vi "createTempControllerFrontEndEvents.vi"(8 "error in (no error)":errorcluster, 11 "CameraEventsManger.lvclass in":refnum<class "CameraEventsManger.lvclass">) -> (0 "error out":errorcluster, 2 "tempControllerFrontEndEvents":T1, 3 "CameraEventsManger.lvclass out":refnum<class "CameraEventsManger.lvclass">)   [LabVIEW 2011, in "Tools.lvlib" / "Settings.lvlib" / "CameraEventsManger.lvclass"]
uses:
  CameraEventsManger.lvclass
  CameraEventsManger.lvclass/CameraEventsManger.ctl
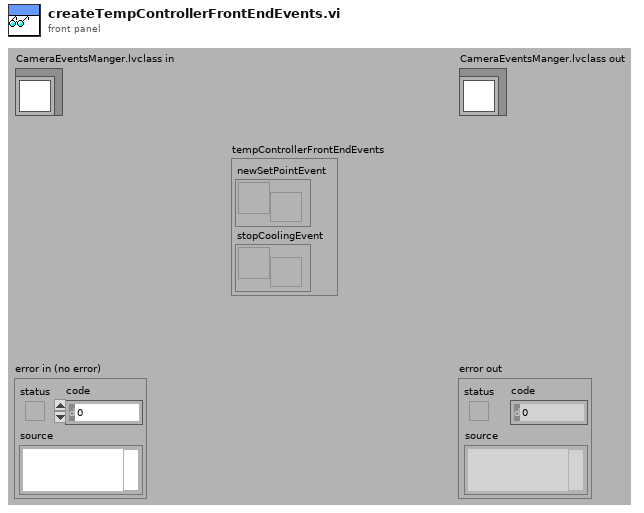
[diagram p1: front panel]
types:
  T1 = cluster{"newSetPointEvent":refnum<user-event>, "stopCoolingEvent":refnum<user-event>}
  T2 = cluster{"newSetPointEvent":cluster{"newSetPoint":i32}, "stopCoolingEvent":cluster{"stopValue":bool}}
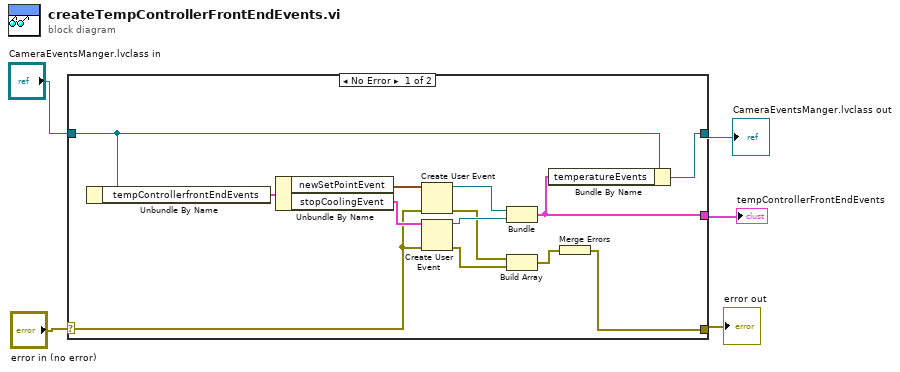
[diagram p0: block diagram]
diagram:
  n1 = case shown="No Error" "error in (no error)" {
    selector: "error in (no error)" -> [w13 w19]
    tunnel: [w9 w19] -> w4
    tunnel: [w7 w20] -> w2
    tunnel: "CameraEventsManger.lvclass in" -> [w8 w20]
    tunnel: [w6 _] -> w1
    frame No Error {
      n2 = Unbundle By Name(w8) -> ("tempControllerfrontEndEvents"=w18:T2)
      n3 = Unbundle By Name(w18) -> ("newSetPointEvent"=w17:cluster{"newSetPoint":i32}, "stopCoolingEvent"=w16:cluster{"stopValue":bool})
      n4 = Create User Event(user event datatype=w17, error in=w13) -> (user event=w14:refnum<user-event>, error out=w11:errorcluster)
      n5 = Create User Event(user event datatype=w16, error in=w13) -> (user event=w15:refnum<user-event>, error out=w10:errorcluster)
      n6 = Bundle("newSetPointEvent"=w14, "stopCoolingEvent"=w15) -> (w6:T1)  [unwired: 1 in]
      n7 = Build Array(w11, w10) -> (w12:errorcluster[])
      n8 = Bundle By Name(cluster=w8, "temperatureEvents"=w6) -> (w7:refnum<class "CameraEventsManger.lvclass">)
      n9 = Merge Errors(w12) -> (w9:errorcluster)
    }
    frame Error {
    }
  }
  "error out" <- w4
  "CameraEventsManger.lvclass out" <- w2
  "tempControllerFrontEndEvents" <- w1
